vi "Notifiers FGV.vi"(8 "error in":errorcluster, 11 "Notifier Action":T1) -> (0 "error out":errorcluster, 3 "ECU Notifiers":T2)   [LabVIEW 2024, in "ECU InterComm.lvlib"]
uses:
  ECU InterComm.lvlib
  ECU Notifiers.ctl
  General Actions.ctl
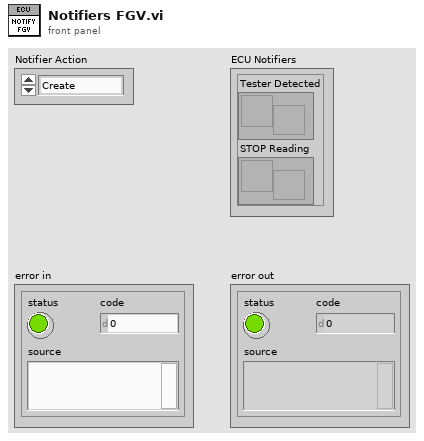
[diagram p1: front panel]
types:
  T1 = typedef "ECU InterComm.lvlib/General Actions.ctl" = enum16{"Create", "Get", "Destroy"}
  T2 = typedef "ECU InterComm.lvlib/ECU Notifiers.ctl" = cluster{"Tester Detected":refnum<notifier>, "STOP Reading":refnum<notifier>}
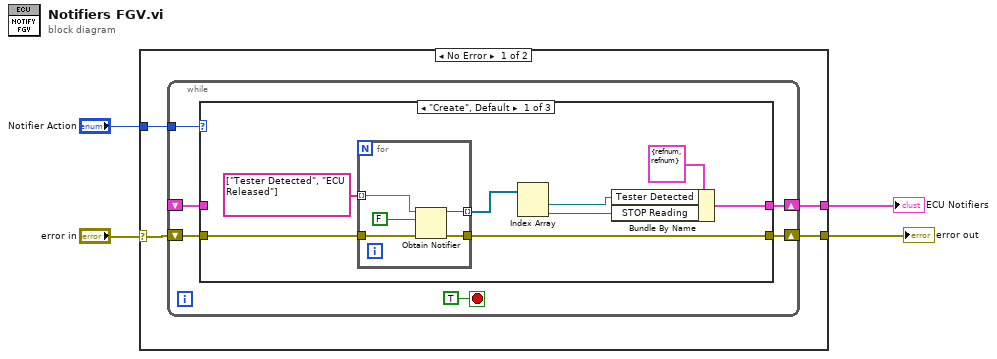
[diagram p0: block diagram]
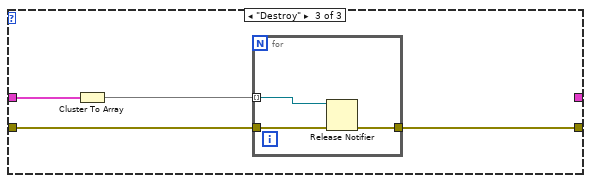
[diagram p3: hidden frame]
diagram:
  n1 = case shown="No Error" "error in" {
    selector: "error in" -> [w5 w37]
    tunnel: "Notifier Action" -> [w8 _]
    tunnel: [w7 _] -> w3
    tunnel: [w6 w37] -> w2
    frame No Error {
      n2 = while {
        tunnel: w8 -> [w13]
        shift-right: [w12] -> w6
        shift-left: w5 -> [w11]
        shift-right: [w10] -> w7
        shift-left: _ -> [w9]
        stop <- TRUE stop-if-true
        n3 = case shown="\"Create\", Default" w13 {
          tunnel: [w22 w29 w32] -> w12
          tunnel: w11 -> [w21 w29 w33]
          tunnel: [w15 w28 _] -> w10
          tunnel: w9 -> [_ w28 w31]
          frame "Create", Default {
            n4 = for {
              tunnel: [w27] -> w22
              tunnel: w21 -> [w26]
              tunnel: string[] ["Tester Detected", "ECU Released"] -> [w25] mode=indexing
              tunnel: [w23] -> w19 mode=indexing
              n5 = Obtain Notifier(name (unnamed)=w25, notification data type=FALSE, error in (no error)=w26) -> (notifier out=w23:refnum<notifier>, error out=w27:errorcluster)  [unwired: 1 in, 1 out]
            }
            n6 = Index Array(array=w19) -> (element #1=w17:refnum<notifier>, element #2=w16:refnum<notifier>)  [unwired: 2 in]
            n7 = Bundle By Name(cluster=T2 {"Tester Detected"=refnum, "STOP Reading"=refnum}, "Tester Detected"=w17, "STOP Reading"=w16) -> (w15:T2)
          }
          frame "Get" {
          }
          frame "Destroy" {
            n8 = Cluster To Array(cluster=w31) -> (array=w30:refnum<notifier>[])
            n9 = for {
              tunnel: w33 -> [w36]
              tunnel: [w35] -> w32
              tunnel: w30 -> [w34] mode=indexing
              n10 = Release Notifier(notifier=w34, error in (no error)=w36) -> (error out=w35:errorcluster)  [unwired: 1 in, 2 out]
            }
          }
        }
      }
    }
    frame Error {
    }
  }
  "ECU Notifiers" <- w3
  "error out" <- w2
